vi "Timer Reset.vi"(8 "error in (no error)":errorcluster, 11 "Timer reference":refnum<data-value>) -> (0 "error out":errorcluster, 3 "Timer reference  out":refnum<data-value>)   [LabVIEW 2018]
doc: "This VI is part of a Timer class that is implemented with the DVR. It resets the Timer and must be called to return the Timer to the 0.\n\nAAL 9/09"
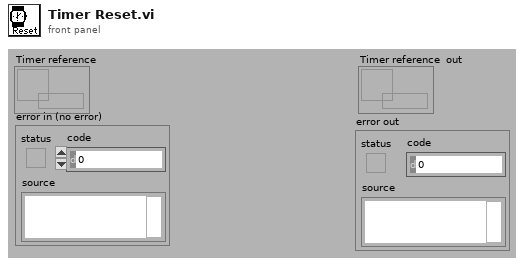
[diagram p1: front panel]
types:
  T1 = cluster{"Start Time":i32, "Elapsed Time":i32, "Running?":bool}
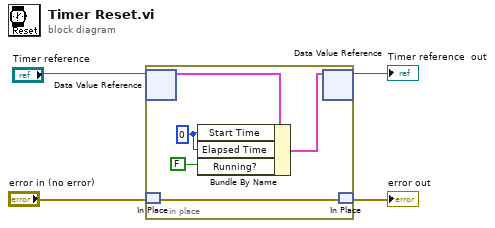
[diagram p0: block diagram]
diagram:
  n1 = in-place {
    w7 = 0 ("Start Time")
    n2 = in-place-dvr #1("Timer reference") -> (w9:T1)  [unwired: 1 out]
    n3 = in-place-match #2("error in (no error)") -> (w5:errorcluster)
    n4 = Bundle By Name(cluster=w9, "Start Time"=w7, "Elapsed Time"=w7, "Running?"=FALSE) -> (w8:T1)
    n5 = in-place-dvr #1(w8) -> (→"Timer reference  out":refnum<data-value>)  [unwired: 1 out]
    n6 = in-place-match #2(w5) -> (→"error out":errorcluster)
  }
